vi "TaskDeinitialize.vi"(8 "error in (no error)":errorcluster, 11 "HGF_Visitable in":refnum<class "HGF_Visitable.lvclass">) -> (0 "error out":errorcluster, 3 "HGF_Visitable out":refnum<class "HGF_Visitable.lvclass">)   [LabVIEW 2014, in "HGF_BaseClasses.lvlib" / "HGF_Visitable.lvclass"]
doc: "Dynamic Dispatch VI.\nCalled by TaskLoop to deinitialize Task"
uses:
  HGF_Visitable.lvclass
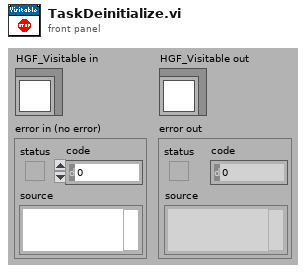
[diagram p1: front panel]
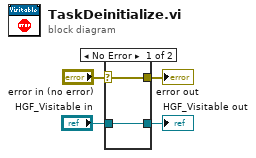
[diagram p0: block diagram]
diagram:
  n1 = case shown="No Error" "error in (no error)" {
    selector: "error in (no error)" -> [w5 w8]
    tunnel: [w5 w8] -> w3
    tunnel: [w6 w7] -> w1
    tunnel: "HGF_Visitable in" -> [w6 w7]
    frame No Error {
    }
    frame Error {
    }
  }
  "error out" <- w3
  "HGF_Visitable out" <- w1
